vi "test.vi"   [LabVIEW 2016]
uses:
  Settings/SettingsTC/TCSettings.lvclass
  home/harini/tcs/ts_sedspectrometer/Settings/Settings/Setting.lvclass
  Settings/ProcessSetting/ProcessSettings.lvclass
  Settings/Settings/Setting.lvclass/Setting.ctl
  Settings/Settings/Setting.lvclass
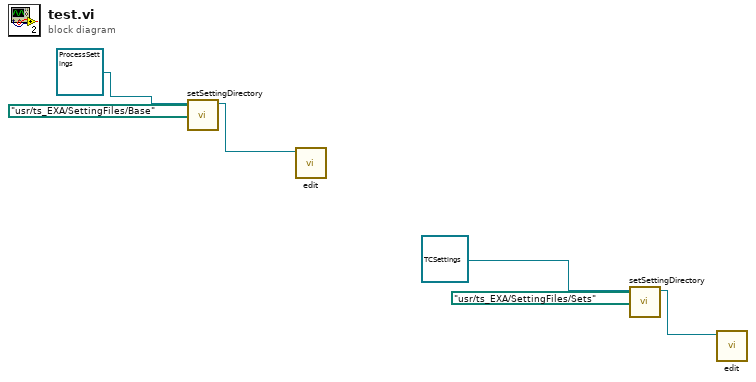
[diagram p0: block diagram]
diagram:
  n1 = call "setSettingDirectory.vi"("SettingDirectory"=path "/usr/ts_EXA/SettingFiles/Base", "BaseSetting in"=refnum<class "ProcessSettings.lvclass"> refnum ("Settings.lvlib:ProcessSettings.lvclass")) -> ("BaseSetting out"=w5:refnum<class "ProcessSettings.lvclass">)  [unwired: 9 in]
  n2 = call-dynamic "edit.vi"("BaseSetting in"=w5) -> ()  [unwired: 8 in, 3 out]
  n3 = call "setSettingDirectory.vi"("SettingDirectory"=path "/usr/ts_EXA/SettingFiles/Sets", "BaseSetting in"=refnum<class "TCSettings.lvclass"> refnum ("Settings.lvlib:TCSettings.lvclass")) -> ("BaseSetting out"=w3:refnum<class "TCSettings.lvclass">)  [unwired: 9 in]
  n4 = call-dynamic "edit.vi"("TCSettings in"=w3) -> ()  [unwired: 8 in, 3 out]
